vi "Test Code - Generating Y Clock Signal.vi"() -> ()   [LabVIEW 2018]
uses:
  <vilib>/DAQmx/create/channels.llb/DAQmx Create Channel (CO-Pulse Generation-Frequency).vi
  <vilib>/DAQmx/configure/timing.llb/DAQmx Timing (Implicit).vi
  <vilib>/DAQmx/configure/timing.llb/DAQmx Timing (Sample Clock).vi
  <resource>/objmgr/daqmx.rc
  <vilib>/Utility/error.llb/DialogType.ctl
  <vilib>/DAQmx/create/channels.llb/DAQmx Create Channel (CI-Count Edges).vi
  <vilib>/DAQmx/read.llb/DAQmx Read (Counter 1D U32 1Chan NSamp).vi
panel:
  out "Laser Clock Error":errorcluster
  out "Y Galvo Error":errorcluster
  out "X Galvo Error":errorcluster
  in  "Stop":bool
  in  "Tab Control":T1(tab)
  in  "Counter Source":tag="Dev1/ctr0"
  in  "Sweep Frequency":dbl=1.0 format="%.6f"
  in  "Sweep Duty Cycle":dbl=0.5 format="%.6f"
  in  "Enable/Disable Sim Laser Clock":bool caption="Enable Sim Laser Clock"
  in  "X Galvo Ch Out":tag="/Dev1/PFI12"
  in  "Enable/Disable X Galvo":bool caption="Enable Galvo"
  in  "Active Edge":i32(ring)=10280 items=["Rising"=10280, "Falling"=10171]
  in  "Trigger Type 2":T2(tab)
  in  "Edge 2":i32(ring)=10280 items=["Rising"=10280, "Falling"=10171]
  in  "Digital Trigger Source 2":tag
  in  "Pause When":i32(ring)=10192 items=["High"=10192, "Low"=10214]
  in  "Pause Trigger Source":tag
  in  "Count Reset Terminal":tag
  in  "Edge 3":i32(ring)=10280 items=["Rising"=10280, "Falling"=10171]
  in  "Input Terminal":tag="PFI8"
  in  "Counter 2":tag="Dev1/ctr0"
  in  "Sample Rate":dbl=1000.0
  in  "Sample Clock Source":tag="PFI0"
  in  "Samples per Loop":i32=100
  out "Data":u32[](array[numeric])
  # "To configure and use a trigger or the count reset you must have the necessary tab selected above.  Not all hardware supports the above options--refer to your device documentation for more info."
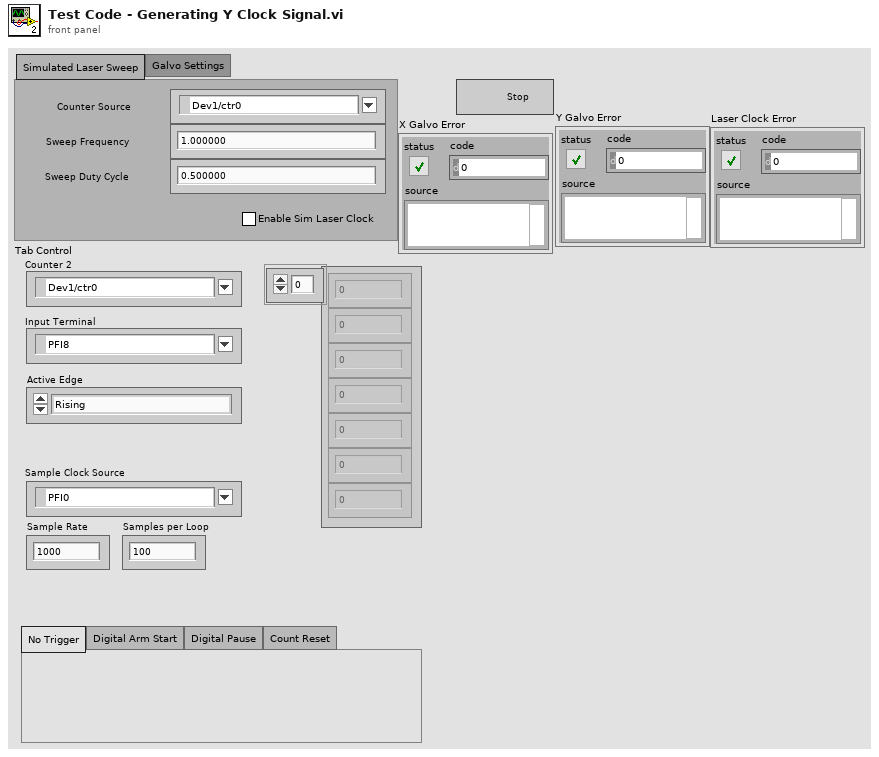
[diagram p1: front panel]
types:
  T1 = enum32{"Simulated Laser Sweep", "Galvo Settings"}
  T2 = enum32{"No Trigger", "Digital Arm Start", "Digital Pause", "Count Reset"}
  T3 = typedef "DialogType.ctl" = u16
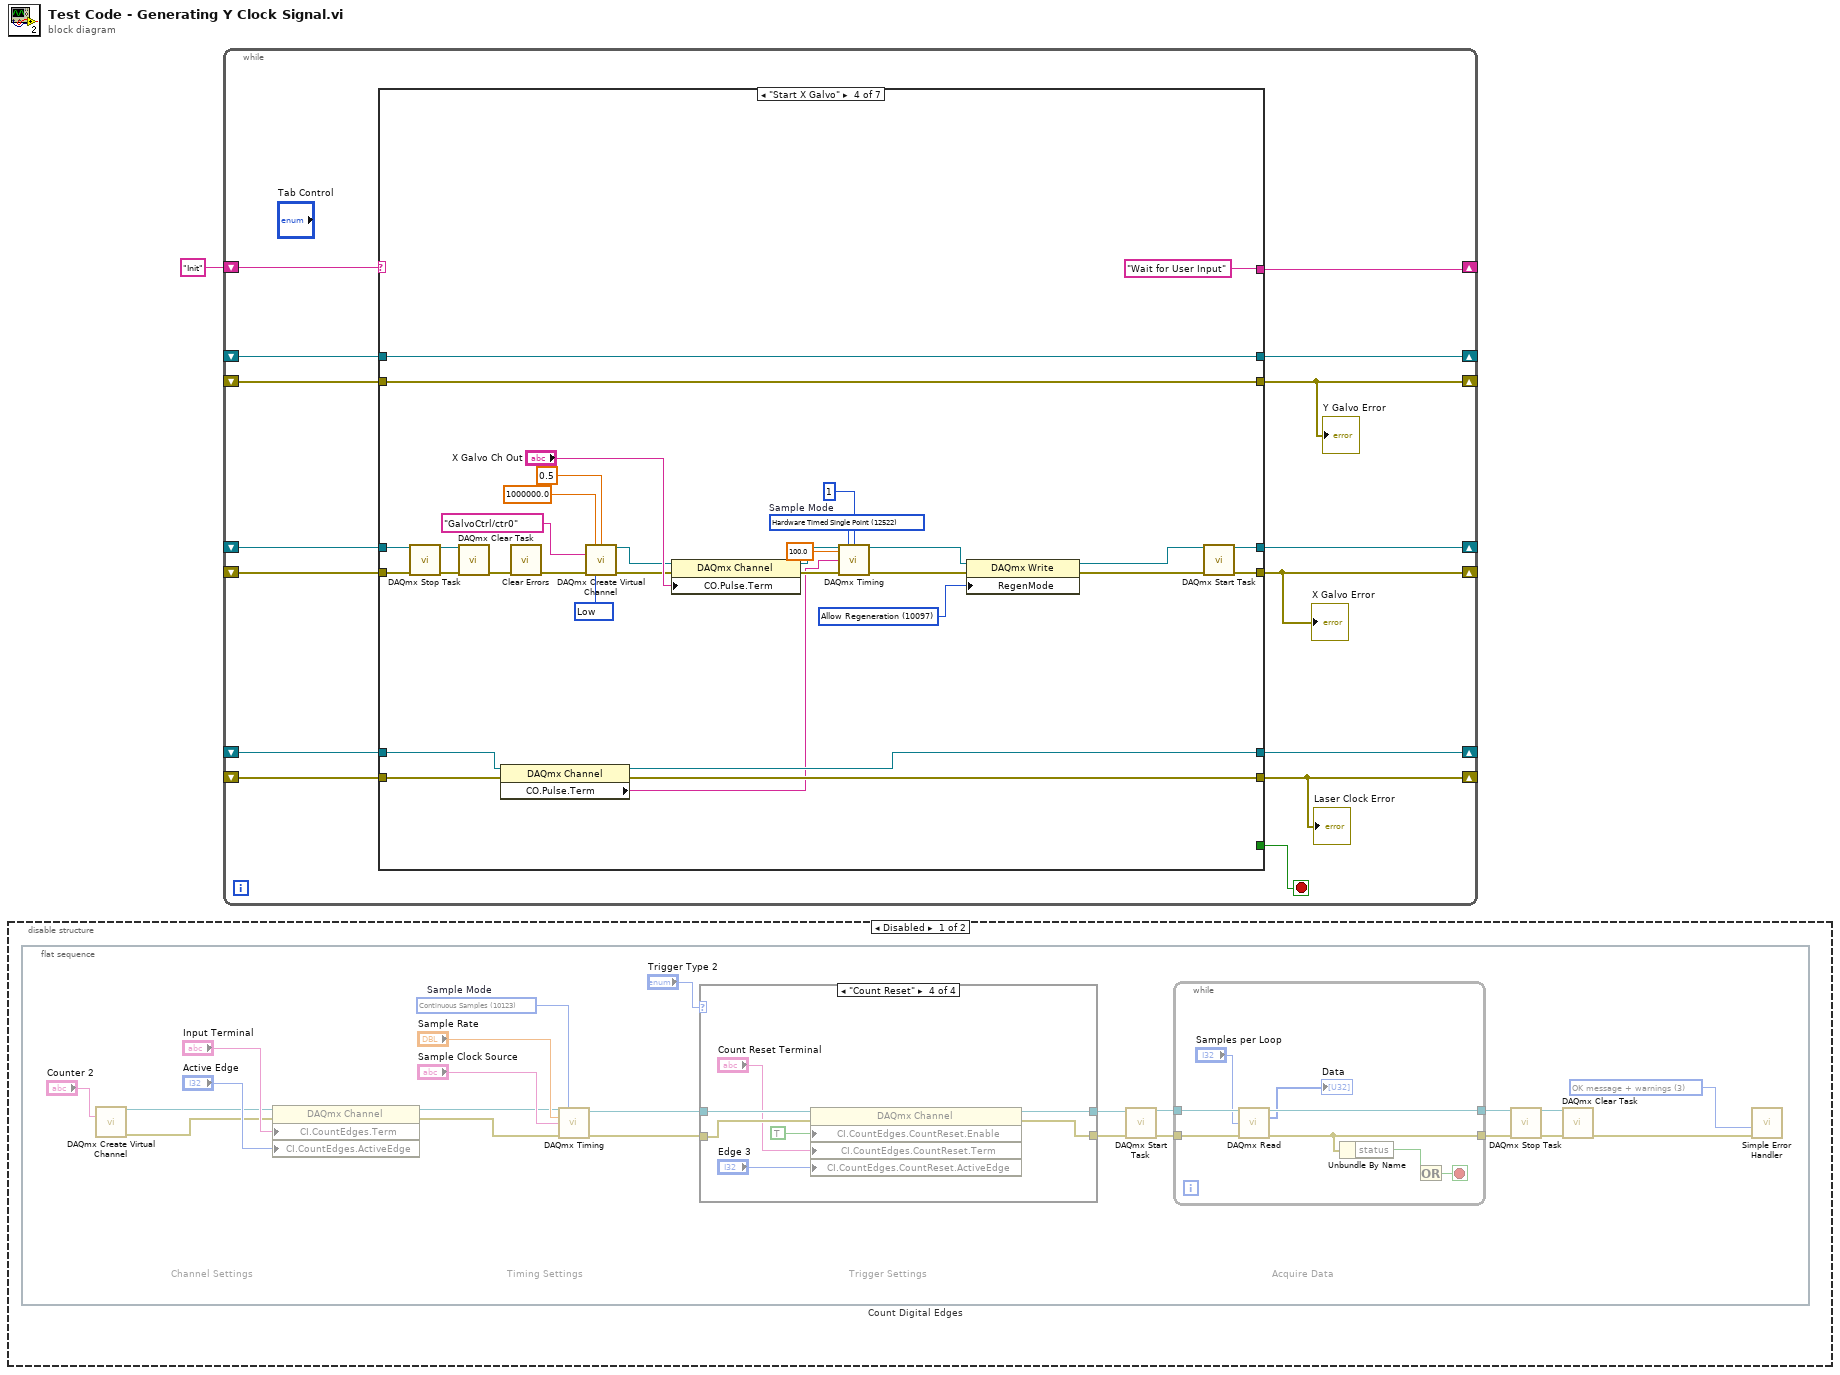
[diagram p0: block diagram]
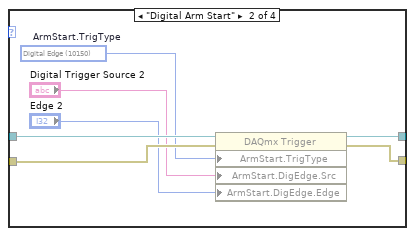
[diagram p3: hidden frame]
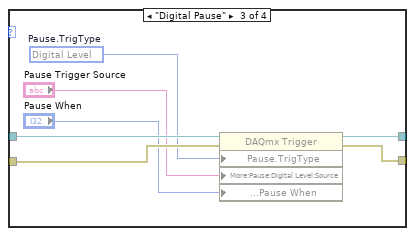
[diagram p4: hidden frame]
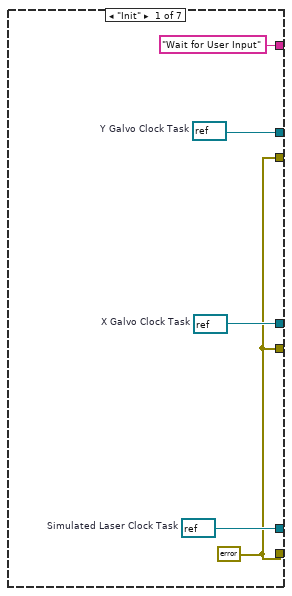
[diagram p6: hidden frame]
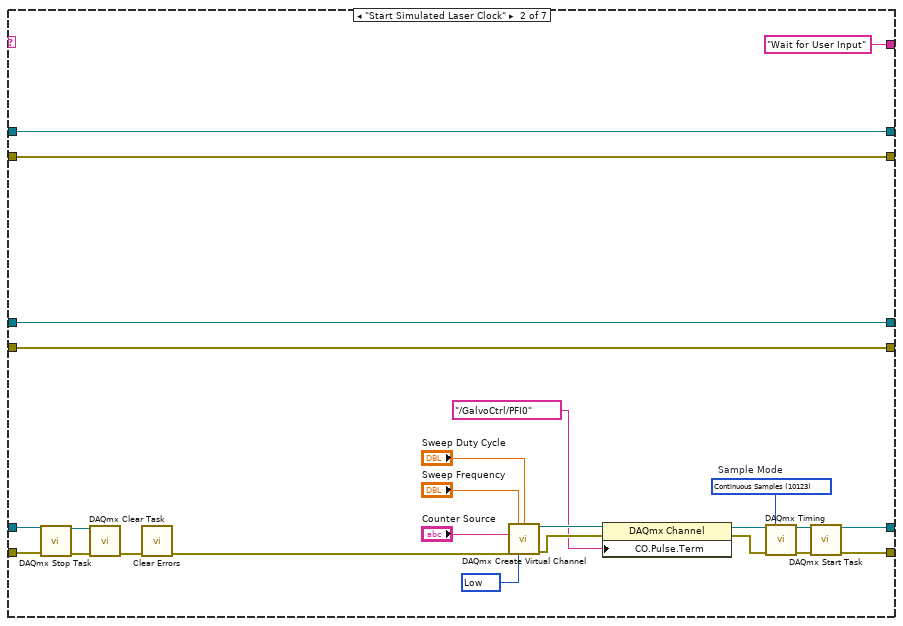
[diagram p7: hidden frame]
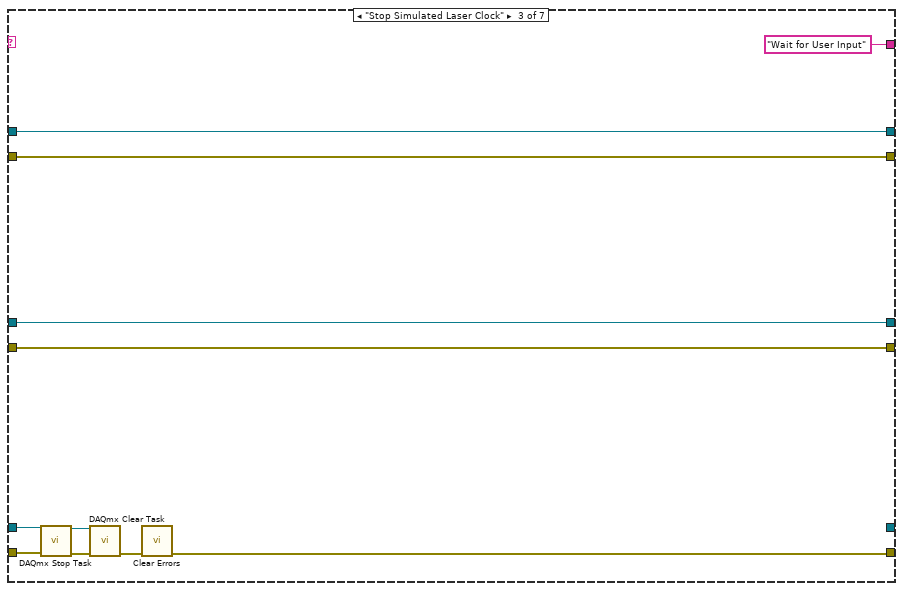
[diagram p8: hidden frame]
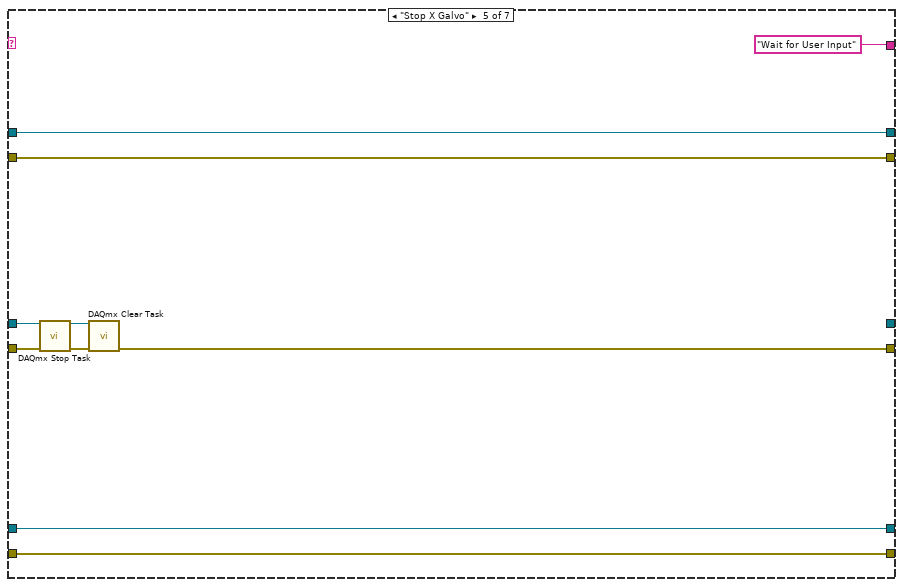
[diagram p9: hidden frame]
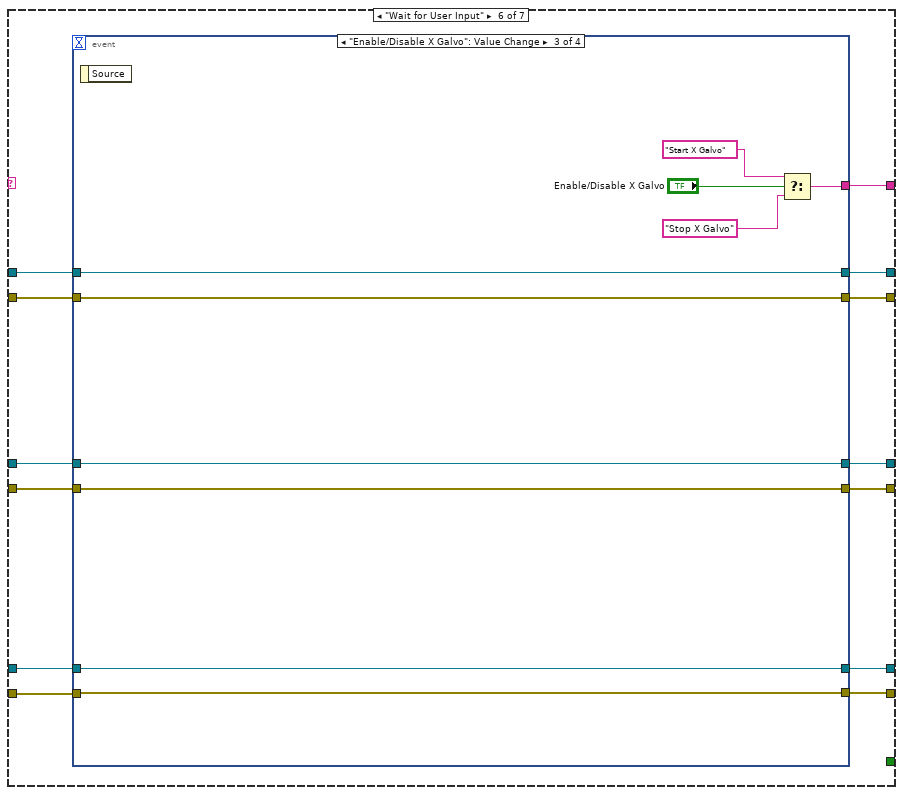
[diagram p10: hidden frame]
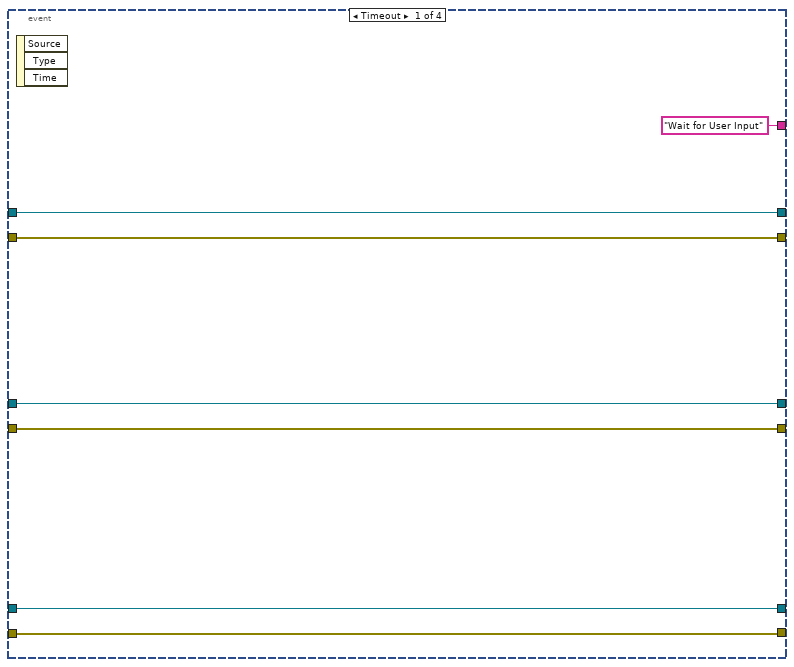
[diagram p11: hidden frame]
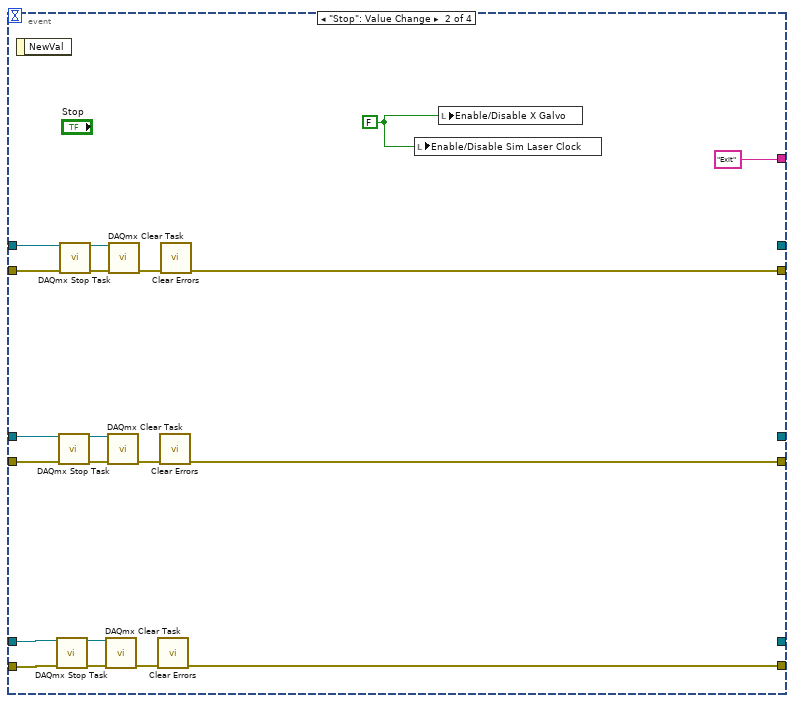
[diagram p12: hidden frame]
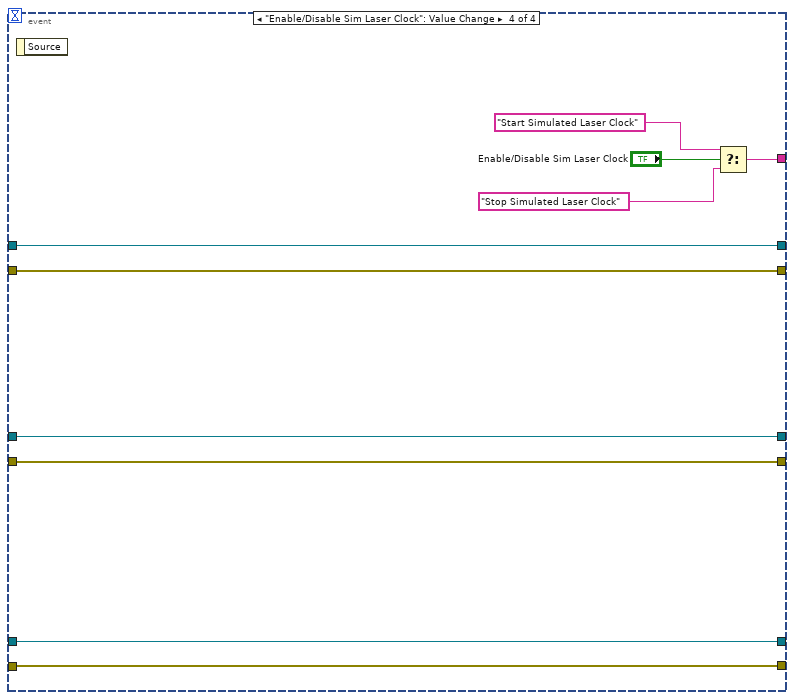
[diagram p13: hidden frame]
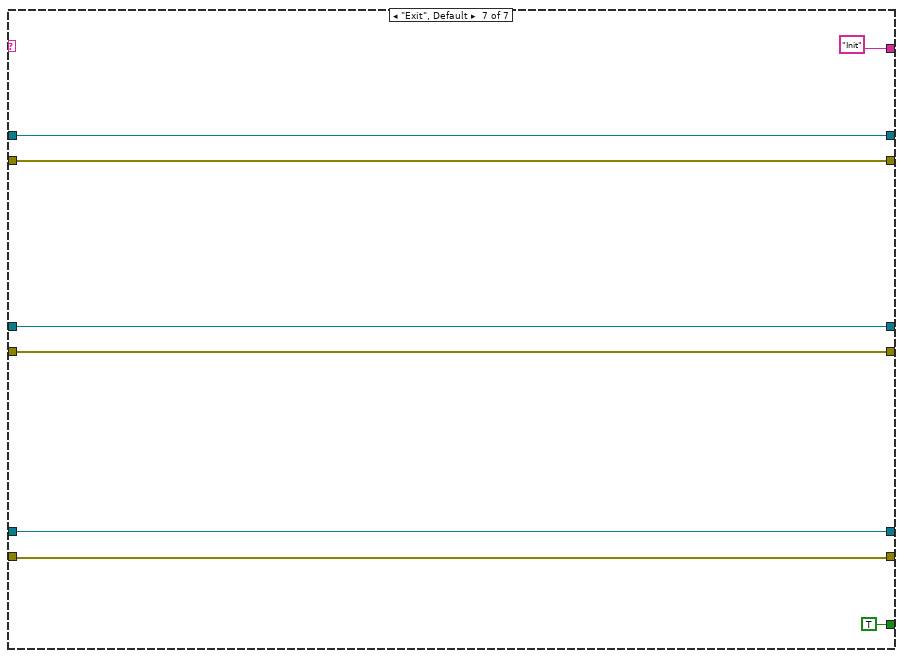
[diagram p14: hidden frame]
diagram:
  n1 = disable-structure shown="Disabled" {
    frame Disabled {
      n2 = flat-sequence "Count Digital Edges" {
        frame #0 {
          w2 = T3 3 items=["no dialog", "OK message", "continue or stop message", "OK message + warnings", "continue/stop + warnings"] ("type of dialog (OK msg:1)")
          w22 = 10123 items=["Finite Samples"=10178, "Continuous Samples"=10123, "Hardware Timed Single Point"=12522]  # Sample Mode
          # "Acquire Data"
          # "Trigger Settings"
          # "Timing Settings"
          # "Channel Settings"
          n3 = call-poly <vilib>:"DAQmx Create Virtual Channel.vi"("counter"="Counter 2") -> ("task out"=w15:refnum<k21>, "error out"=w12:errorcluster)  [unwired: 13 in]
          n4 = property class="DAQmx Channel"(reference=w15, error in=w12, "CI.CountEdges.Term"="Input Terminal", "CI.CountEdges.ActiveEdge"="Active Edge") -> (reference out=w14:refnum<k21>, error out=w13:errorcluster)
          n5 = call-poly <vilib>:"DAQmx Timing.vi"("task/channels in"=w14, "sample mode"=w22, "rate"="Sample Rate", "source"="Sample Clock Source", "error in"=w13) -> ("task out"=w8:refnum<k21>, "error out"=w7:errorcluster)  [unwired: 9 in]
          n6 = case shown="\"Count Reset\"" "Trigger Type 2" {
            tunnel: w8 -> [w26 w33 w40 w47]
            tunnel: w7 -> [w25 w30 w37 w44]
            tunnel: [w26 w32 w39 w46] -> w9
            tunnel: [w25 w31 w38 w45] -> w10
            frame "No Trigger", Default {
            }
            frame "Digital Arm Start" {
              w27 = 10150 items=["Digital Edge"=10150, "None"=10230]  # ArmStart.TrigType
              n7 = property class="DAQmx Trigger"(reference=w33, error in=w30, "ArmStart.TrigType"=w27, "ArmStart.DigEdge.Src"="Digital Trigger Source 2", "ArmStart.DigEdge.Edge"="Edge 2") -> (reference out=w32:refnum<k21>, error out=w31:errorcluster)
            }
            frame "Digital Pause" {
              w36 = 10152 items=["Analog Level"=10101, "Analog Window"=10103, "Digital Level"=10152, "Digital Pattern"=10398, "None"=10230]  # Pause.TrigType
              n8 = property class="DAQmx Trigger"(reference=w40, error in=w37, "Pause.TrigType"=w36, "More:Pause:Digital Level:Source"="Pause Trigger Source", "More:Pause:Digital Level:Pause When"="Pause When") -> (reference out=w39:refnum<k21>, error out=w38:errorcluster)
            }
            frame "Count Reset" {
              n9 = property class="DAQmx Channel"(reference=w47, error in=w44, "CI.CountEdges.CountReset.Enable"=TRUE, "CI.CountEdges.CountReset.Term"="Count Reset Terminal", "CI.CountEdges.CountReset.ActiveEdge"="Edge 3") -> (reference out=w46:refnum<k21>, error out=w45:errorcluster)
            }
          }
          n10 = call <vilib>:"DAQmx Start Task.vi"("task/channels in"=w9, "error in"=w10) -> ("task out"=w21:refnum<k21>, "error out"=w20:errorcluster)  [unwired: 12 in]
          n11 = while {
            tunnel: w21 -> [w56]
            tunnel: w20 -> [w55]
            tunnel: [w52] -> w5
            tunnel: [w53] -> w6
            stop <- w54 stop-if-true
            n12 = call-poly <vilib>:"DAQmx Read.vi"("task/channels in"=w56, "number of samples per channel"="Samples per Loop", "error in"=w55) -> ("task out"=w53:refnum<k21>, "data"=→"Data":u32[], "error out"=w52:errorcluster)  [unwired: 10 in]
            n13 = Unbundle By Name(w52) -> ("status"=w51:bool)
            n14 = Or(x=w51) -> (y=w49:bool, x .or. y?=w54:bool)
          }
          n15 = call <vilib>:"DAQmx Stop Task.vi"("task/channels in"=w6, "error in"=w5) -> ("task out"=w3:refnum<k21>, "error out"=w4:errorcluster)  [unwired: 12 in]
          n16 = call <vilib>:"DAQmx Clear Task.vi"("task in"=w3, "error in"=w4) -> ("error out"=w19:errorcluster)  [unwired: 13 in]
          n17 = call <vilib>:"Simple Error Handler.vi"("type of dialog (OK msg:1)"=w2, "error in (no error)"=w19) -> ()  [unwired: 3 in, 5 out]
        }
      }
    }
    frame Enabled {
    }
  }
  n18 = while {
    shift-right: [w69] -> _
    shift-left: "Init" -> [w70]
    shift-right: [w68] -> _
    shift-left: _ -> [w67]
    shift-right: [w57] -> _
    shift-left: _ -> [w66]
    shift-right: [w65] -> _
    shift-left: _ -> [w63]
    shift-right: [w64] -> _
    shift-left: _ -> [w62]
    shift-right: [w61] -> _
    shift-left: _ -> [w60]
    shift-right: [w58] -> _
    shift-left: _ -> [w59]
    stop <- w71 stop-if-true
    n19 = case shown="\"Start X Galvo\"" w70 {
      tunnel: [_ _ _ _ _ _ TRUE] -> w71
      tunnel: ["Wait for User Input" "Wait for User Input" "Wait for User Input" "Wait for User Input" "Wait for User Input" w168 "Init"] -> w69
      tunnel: [w75 w89 _ w123 w152 w164 w220] -> w68
      tunnel: w67 -> [_ w84 w109 w124 w152 w167 w220]
      tunnel: [w72 w88 w102 w125 w151 w165 w221] -> w57
      tunnel: w66 -> [_ w85 w110 w126 w151 w166 w221]
      tunnel: [w74 w80 w106 w128 _ w157 w219] -> w65
      tunnel: [w73 w78 w104 w145 w155 w156 w218] -> w64
      tunnel: w63 -> [_ w80 w106 w134 w147 w163 w219]
      tunnel: w62 -> [_ w78 w104 w145 w155 w162 w218]
      tunnel: [w72 w81 w107 w130 w146 w161 w216] -> w61
      tunnel: w60 -> [_ w81 w107 w135 w148 w160 w216]
      tunnel: [w72 w79 w105 w144 w154 w159 w217] -> w58
      tunnel: w59 -> [_ w79 w105 w144 w154 w158 w217]
      frame "Init" {
        w73 = refnum<k21> refnum  # Y Galvo Clock Task
        w74 = refnum<k21> refnum  # X Galvo Clock Task
        w72 = errorcluster {"status"=FALSE, "code"=0, "source"=""} ("error out")
        w75 = refnum<k21> refnum  # Simulated Laser Clock Task
      }
      frame "Start Simulated Laser Clock" {
        w90 = 10214 items=["High"=10192, "Low"=10214] ("idle state")
        w91 = 10123 items=["Finite Samples"=10178, "Continuous Samples"=10123, "Hardware Timed Single Point"=12522]  # Sample Mode
        n20 = call <vilib>:"DAQmx Stop Task.vi"("task/channels in"=w84, "error in"=w85) -> ("task out"=w86:refnum<k21>, "error out"=w87:errorcluster)  [unwired: 12 in]
        n21 = call <vilib>:"DAQmx Clear Task.vi"("task in"=w86, "error in"=w87) -> ("error out"=w83:errorcluster)  [unwired: 13 in]
        n22 = call <vilib>:"Clear Errors.vi"("error in (no error)"=w83) -> ("error out"=w82:errorcluster)  [unwired: 5 in, 1 out]
        n23 = call-poly <vilib>:"DAQmx Create Virtual Channel.vi"("frequency"="Sweep Frequency", "duty cycle"="Sweep Duty Cycle", "counter"="Counter Source", "error in"=w82, "idle state"=w90) -> ("task out"=w96:refnum<k21>, "error out"=w97:errorcluster)  [unwired: 9 in]
        n24 = property class="DAQmx Channel"(reference=w96, error in=w97, "CO.Pulse.Term"=tag "/GalvoCtrl/PFI0" ("Output Terminal 2")) -> (reference out=w99:refnum<k21>, error out=w98:errorcluster)
        n25 = call-poly <vilib>:"DAQmx Timing.vi"("task/channels in"=w99, "sample mode"=w91, "error in"=w98) -> ("task out"=w95:refnum<k21>, "error out"=w94:errorcluster)  [unwired: 11 in]
        n26 = call <vilib>:"DAQmx Start Task.vi"("task/channels in"=w95, "error in"=w94) -> ("task out"=w89:refnum<k21>, "error out"=w88:errorcluster)  [unwired: 12 in]
      }
      frame "Stop Simulated Laser Clock" {
        n27 = call <vilib>:"DAQmx Stop Task.vi"("task/channels in"=w109, "error in"=w110) -> ("task out"=w111:refnum<k21>, "error out"=w112:errorcluster)  [unwired: 12 in]
        n28 = call <vilib>:"DAQmx Clear Task.vi"("task in"=w111, "error in"=w112) -> ("error out"=w108:errorcluster)  [unwired: 13 in]
        n29 = call <vilib>:"Clear Errors.vi"("error in (no error)"=w108) -> ("error out"=w102:errorcluster)  [unwired: 5 in, 1 out]
      }
      frame "Start X Galvo" {
        w122 = 10097 items=["Allow Regeneration"=10097, "Do Not Allow Regeneration"=10158] ("RegenMode")
        w127 = 10214 items=["High"=10192, "Low"=10214] ("idle state")
        w132 = 12522 items=["Finite Samples"=10178, "Continuous Samples"=10123, "Hardware Timed Single Point"=12522]  # Sample Mode
        n30 = call <vilib>:"DAQmx Stop Task.vi"("task/channels in"=w134, "error in"=w135) -> ("task out"=w137:refnum<k21>, "error out"=w138:errorcluster)  [unwired: 12 in]
        n31 = call <vilib>:"DAQmx Clear Task.vi"("task in"=w137, "error in"=w138) -> ("error out"=w136:errorcluster)  [unwired: 13 in]
        n32 = property class="DAQmx Channel"(reference=w124, error in=w126) -> (reference out=w123:refnum<k21>, error out=w125:errorcluster, "CO.Pulse.Term"=w116:tag)
        n33 = call <vilib>:"Clear Errors.vi"("error in (no error)"=w136) -> ("error out"=w133:errorcluster)  [unwired: 5 in, 1 out]
        n34 = call-poly <vilib>:"DAQmx Create Virtual Channel.vi"("frequency"=1000000.0, "duty cycle"=0.5, "counter"=tag "GalvoCtrl/ctr0" ("Counter 3"), "error in"=w133, "idle state"=w127) -> ("task out"=w140:refnum<k21>, "error out"=w141:errorcluster)  [unwired: 9 in]
        n35 = property class="DAQmx Channel"(reference=w140, error in=w141, "CO.Pulse.Term"="X Galvo Ch Out") -> (reference out=w129:refnum<k21>, error out=w131:errorcluster)
        n36 = call-poly <vilib>:"DAQmx Timing.vi"("task/channels in"=w129, "sample mode"=w132, "samples per channel"=1, "rate"=100.0, "source"=w116, "error in"=w131) -> ("task out"=w119:refnum<k21>, "error out"=w120:errorcluster)  [unwired: 8 in]
        n37 = property class="DAQmx Write"(reference=w119, error in=w120, "RegenMode"=w122) -> (reference out=w117:refnum<k21>, error out=w118:errorcluster)
        n38 = call <vilib>:"DAQmx Start Task.vi"("task/channels in"=w117, "error in"=w118) -> ("task out"=w128:refnum<k21>, "error out"=w130:errorcluster)  [unwired: 12 in]
      }
      frame "Stop X Galvo" {
        n39 = call <vilib>:"DAQmx Stop Task.vi"("task/channels in"=w147, "error in"=w148) -> ("task out"=w149:refnum<k21>, "error out"=w150:errorcluster)  [unwired: 12 in]
        n40 = call <vilib>:"DAQmx Clear Task.vi"("task in"=w149, "error in"=w150) -> ("error out"=w146:errorcluster)  [unwired: 13 in]
      }
      frame "Wait for User Input" {
        n41 = event shown="[2] \"Enable/Disable X Galvo\": Value Change" {
          selector: _ -> [_ _ _ _]
          dyn-events: _ -> [_ _ _ _]
          timeout: _ -> [_ _ _ _]
          tunnel: ["Wait for User Input" "Exit" w199 w209] -> w168
          tunnel: w167 -> [w174 w190 w201 w211]
          tunnel: w166 -> [w175 w191 w200 w210]
          tunnel: [w175 w189 w200 w210] -> w165
          tunnel: [w174 _ w201 w211] -> w164
          tunnel: w163 -> [w170 w182 w203 w213]
          tunnel: w162 -> [w169 w181 w205 w215]
          tunnel: [w172 w180 w202 w212] -> w161
          tunnel: w160 -> [w172 w179 w202 w212]
          tunnel: [w171 w178 w204 w214] -> w159
          tunnel: w158 -> [w171 w177 w204 w214]
          tunnel: [w170 _ w203 w213] -> w157
          tunnel: [w169 _ w205 w215] -> w156
          event Timeout {
            n42 = event-data() -> ()  [unwired: 1 in, 3 out]
          }
          event "Stop": Value Change {
            w176 = FALSE
            n43 = event-data() -> ()  [unwired: 1 in, 1 out]
            n44 = call <vilib>:"DAQmx Stop Task.vi"("task/channels in"=w190, "error in"=w191) -> ("task out"=w193:refnum<k21>, "error out"=w194:errorcluster)  [unwired: 12 in]
            n45 = call <vilib>:"DAQmx Stop Task.vi"("task/channels in"=w182, "error in"=w179) -> ("task out"=w187:refnum<k21>, "error out"=w186:errorcluster)  [unwired: 12 in]
            n46 = call <vilib>:"DAQmx Stop Task.vi"("task/channels in"=w181, "error in"=w177) -> ("task out"=w184:refnum<k21>, "error out"=w185:errorcluster)  [unwired: 12 in]
            n47 = call <vilib>:"DAQmx Clear Task.vi"("task in"=w193, "error in"=w194) -> ("error out"=w192:errorcluster)  [unwired: 13 in]
            n48 = call <vilib>:"DAQmx Clear Task.vi"("task in"=w187, "error in"=w186) -> ("error out"=w188:errorcluster)  [unwired: 13 in]
            n49 = call <vilib>:"DAQmx Clear Task.vi"("task in"=w184, "error in"=w185) -> ("error out"=w183:errorcluster)  [unwired: 13 in]
            n50 = call <vilib>:"Clear Errors.vi"("error in (no error)"=w192) -> ("error out"=w189:errorcluster)  [unwired: 5 in, 1 out]
            n51 = call <vilib>:"Clear Errors.vi"("error in (no error)"=w188) -> ("error out"=w180:errorcluster)  [unwired: 5 in, 1 out]
            n52 = call <vilib>:"Clear Errors.vi"("error in (no error)"=w183) -> ("error out"=w178:errorcluster)  [unwired: 5 in, 1 out]
            n53 = local write "Enable/Disable Sim Laser Clock"(w176) -> ()
            n54 = local write "Enable/Disable X Galvo"(w176) -> ()
          }
          event "Enable/Disable X Galvo": Value Change {
            n55 = event-data() -> ()  [unwired: 1 in, 1 out]
            n56 = Select(t="Start X Galvo", s="Enable/Disable X Galvo", f="Stop X Galvo") -> (s? t:f=w199:string)
          }
          event "Enable/Disable Sim Laser Clock": Value Change {
            n57 = event-data() -> ()  [unwired: 1 in, 1 out]
            n58 = Select(t="Start Simulated Laser Clock", s="Enable/Disable Sim Laser Clock", f="Stop Simulated Laser Clock") -> (s? t:f=w209:string)
          }
        }
      }
      frame "Exit", Default {
      }
    }
    "X Galvo Error" <- w61
    "Y Galvo Error" <- w58
    "Laser Clock Error" <- w57
  }
